vi "ARCH_EDITOR_records_click_discard.vi"(10 "CellPosition":T2, 11 "event_structure_shift_register_in":T1={"REF_EDIT_clicked_row"=-1, "REF_EDIT_selected_row"=-1, "SQL_EDIT_clicked_row"=-1, "SQL_EDIT_selected_row"=-1, "ARCH_EDIT_selected_row"=-1, "ARCH_EDIT_clicked_row"=-1, "USER_EDIT_selected_row"=-1, "USER_EDIT_clicked_row"=-1, "REPORT_GEAR_toggle_all_results"=FALSE}) -> (2 "Discard?":bool, 3 "event_structure_shift_register_out":T1={"REF_EDIT_clicked_row"=-1, "REF_EDIT_selected_row"=-1, "SQL_EDIT_clicked_row"=-1, "SQL_EDIT_selected_row"=-1, "ARCH_EDIT_selected_row"=-1, "ARCH_EDIT_clicked_row"=-1, "USER_EDIT_selected_row"=-1, "USER_EDIT_clicked_row"=-1, "REPORT_GEAR_toggle_all_results"=FALSE})   [LabVIEW 2019]
uses:
  CLIENT_event_structure_shift_register.ctl
  <vilib>/Utility/miscctls.llb/LVRowAndColumnTypeDef.ctl
  FGV/ARCH_EDITOR_records_display/FGV_ARCH_EDITOR_records_display.ctl
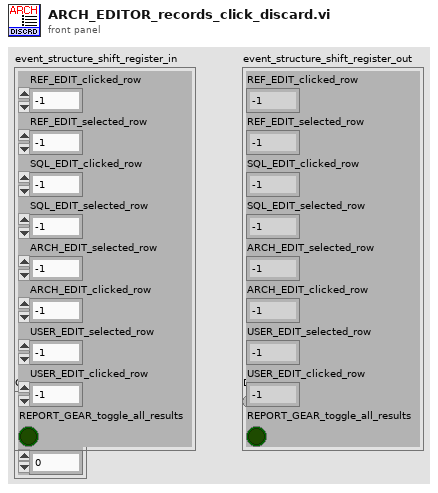
[diagram p1: front panel]
types:
  T1 = typedef "CLIENT_event_structure_shift_register.ctl" = cluster{"REF_EDIT_clicked_row":i32, "REF_EDIT_selected_row":i32, "SQL_EDIT_clicked_row":i32, "SQL_EDIT_selected_row":i32, "ARCH_EDIT_selected_row":i32, "ARCH_EDIT_clicked_row":i32, "USER_EDIT_selected_row":i32, "USER_EDIT_clicked_row":i32, "REPORT_GEAR_toggle_all_results":bool}
  T2 = typedef "LVRowAndColumnTypeDef.ctl" = cluster{"Row":i32, "Column":i32}
  T3 = typedef "FGV_ARCH_EDITOR_records_display.ctl" = enum16{"initialize", "set_arch_cfg_tables_names", "set_station_number", "set_type_filter", "set_headers", "set_records", "get_arch_cfg_table_name", "get_arch_cfg_hist_table_name", "get_station_number", "get_type_filter", "get_headers", "get_uneditable_columns", "get_all_info", "record_added?", "record_inserted?", "record_edited?", "record_updated?", "record_deleted?", "discard_changes"}
  T4 = typedef "ARCH_EDITOR_all_info.ctl" = cluster{"station_number":string, "type_filter":string, "archivisation_cfg_table":string, "archivisation_cfg_history":string, "column_names":string[], "uneditable_columns":string[], "uneditable_columns":i32[], "editable_columns":i32[], "values_in_database":string[][], "size":cluster{"columns":i32, "SQL_rows":i32, "disp_rows":i32}, "ARCH_record_states":T5[]}
  T5 = typedef "SQL_record_states.ctl" = enum16{"Equal", "Added", "Edited", "Deleted"}
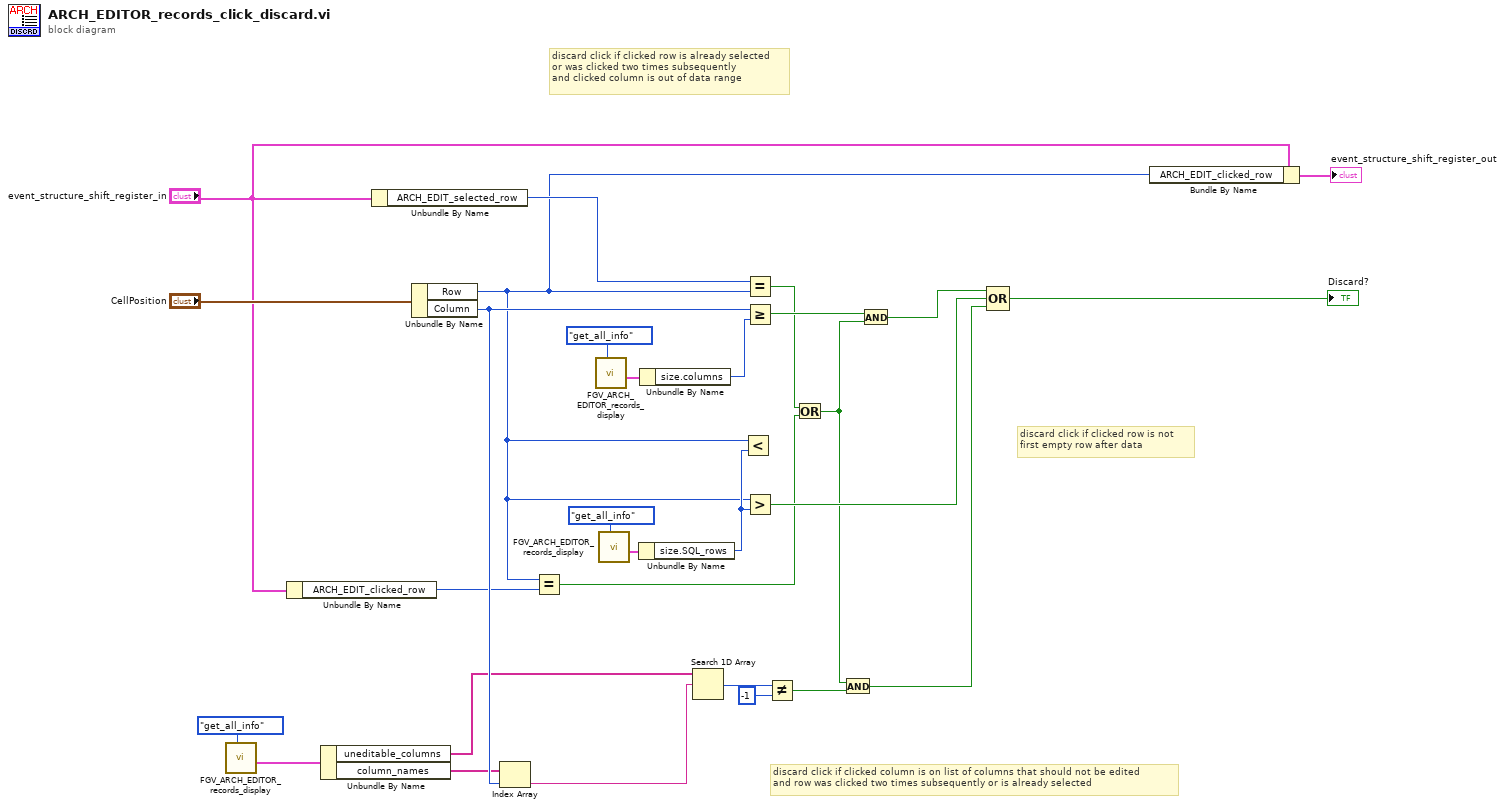
[diagram p0: block diagram]
diagram:
  # "discard click if clicked column is on list of columns that should not be edited\nand row was clicked two times subsequently or is already selected"
  # "discard click if clicked row is not \nfirst empty row after data"
  # "discard click if clicked row is already selected\nor was clicked two times subsequently\nand clicked column is out of data range"
  n1 = call "FGV_ARCH_EDITOR_records_display.vi"("options"=FGV_ARCH_EDITOR_records_display."get_all_info") -> ("all_info"=w4:T4)  [unwired: 7 in, 3 out]
  n2 = Unbundle By Name("event_structure_shift_register_in") -> ("ARCH_EDIT_clicked_row"=w10:i32)
  n3 = Unbundle By Name(w4) -> ("uneditable_columns"=w2:string[], "column_names"=w3:string[])
  n4 = Unbundle By Name("event_structure_shift_register_in") -> ("ARCH_EDIT_selected_row"=w14:i32)
  n5 = Unbundle By Name("CellPosition") -> ("Row"=w9:i32, "Column"=w22:i32)
  n6 = Index Array(array=w3, index=w22) -> (element=w21:string)
  n7 = Equal?(x=w9, y=w10) -> (x = y?=w6:bool)
  n8 = call "FGV_ARCH_EDITOR_records_display.vi"("options"=FGV_ARCH_EDITOR_records_display."get_all_info") -> ("all_info"=w26:T4)  [unwired: 7 in, 3 out]
  n9 = call "FGV_ARCH_EDITOR_records_display.vi"("options"=FGV_ARCH_EDITOR_records_display."get_all_info") -> ("all_info"=w28:T4)  [unwired: 7 in, 3 out]
  n10 = Unbundle By Name(w28) -> ("size.SQL_rows"=w13:i32)
  n11 = Unbundle By Name(w26) -> ("size.columns"=w25:i32)
  n12 = Search 1D Array(1D array=w2, element=w21) -> (index of element=w20:i32)  [unwired: 1 in]
  n13 = Less?(x=w9, y=w13) -> ()  [unwired: 1 out]
  n14 = Equal?(x=w14, y=w9) -> (x = y?=w7:bool)
  n15 = Greater Or Equal?(x=w22, y=w25) -> (x >= y?=w8:bool)
  n16 = Greater?(x=w9, y=w13) -> (0:w15:bool)
  n17 = Not Equal?(x=w20, y=-1) -> (x != y?=w12:bool)
  n18 = Or(x=w7, y=w6) -> (x .or. y?=w5:bool)
  n19 = And(x=w5, y=w12) -> (x .and. y?=w17:bool)
  n20 = And(x=w8, y=w5) -> (x .and. y?=w18:bool)
  n21 = Compound Arithmetic op=OR(w18, w15, w17) -> (→"Discard?":bool)
  n22 = Bundle By Name(cluster="event_structure_shift_register_in", "ARCH_EDIT_clicked_row"=w9) -> (→"event_structure_shift_register_out":T1)
